vi "U3 DAC_Kevin_MFC_PID.vi"() -> ()   [LabVIEW 2016]
uses:
  OdorSensorArray/labview 2016 code/osa_global_save2.vi
  <vilib>/Utility/file.llb/Read From Spreadsheet File (DBL).vi
  <vilib>/measure/NI_MABase.lvlib
panel:
  out "Error  PID_Save":string
  out "error write":errorcluster
  in  "Save file":bool
  in  "data folder":path
  out "appended path":path
  out "PID_read":dbl(graph)
  out "AIN0":dbl format="%.6f"
  out "MFC I/O":cluster{"Value Read":dbl, "Value Read":dbl}(graph)
  out "AIN2":dbl format="%.6f"
  out "AIN1":dbl format="%.6f"
  in  "DAC0_type":enum16{"functional", "fixed", "read"}(ring)
  out "Array Size":i32
  out "Udate Array from File":sgl[](array[numeric])
  out "Waveform Chart":dbl(graph)
  in  "DAC0_fixed":dbl step=0.1 format="%.4f"
  out "Error DAC1,B":string
  out "error read":errorcluster
  in  "DAC1&DACB_fixed":dbl step=0.1 format="%.4f"
  in  "Update Interval (ms)":u32=20
  out "Error_DAC0":string
  in  "Function":u16(ring) items=["Sine Wave", "Triangle Wave", "Square Wave", "Sawtooth Wave"]
  in  "Min Voltage":dbl=0.5 min=0.0 max=5.0 step=0.1 format="%.2f"
  in  "Max Voltage":dbl=4.5 min=0.0 max=5.0 step=0.1 format="%.2f"
  in  "Frequency (Hz)":dbl=1.0 step=0.1 format="%.3f"
  in  "Stop":bool
  # "Updates DAC0 at the specified update interval in order to build time series waveforms.  The\nupdate interval is set to 20 ms by default, but can be set lower based on the execution times\ndiscussed in Section 3.1 of the U3 User's Guide.  Uses the first found U3.\n\nWith a software timed application such as this, you might be able to reduce timing jitter (caused\nby the operating system) by increasing the priority of this process (labview.exe) in Windows\nTask Manager."
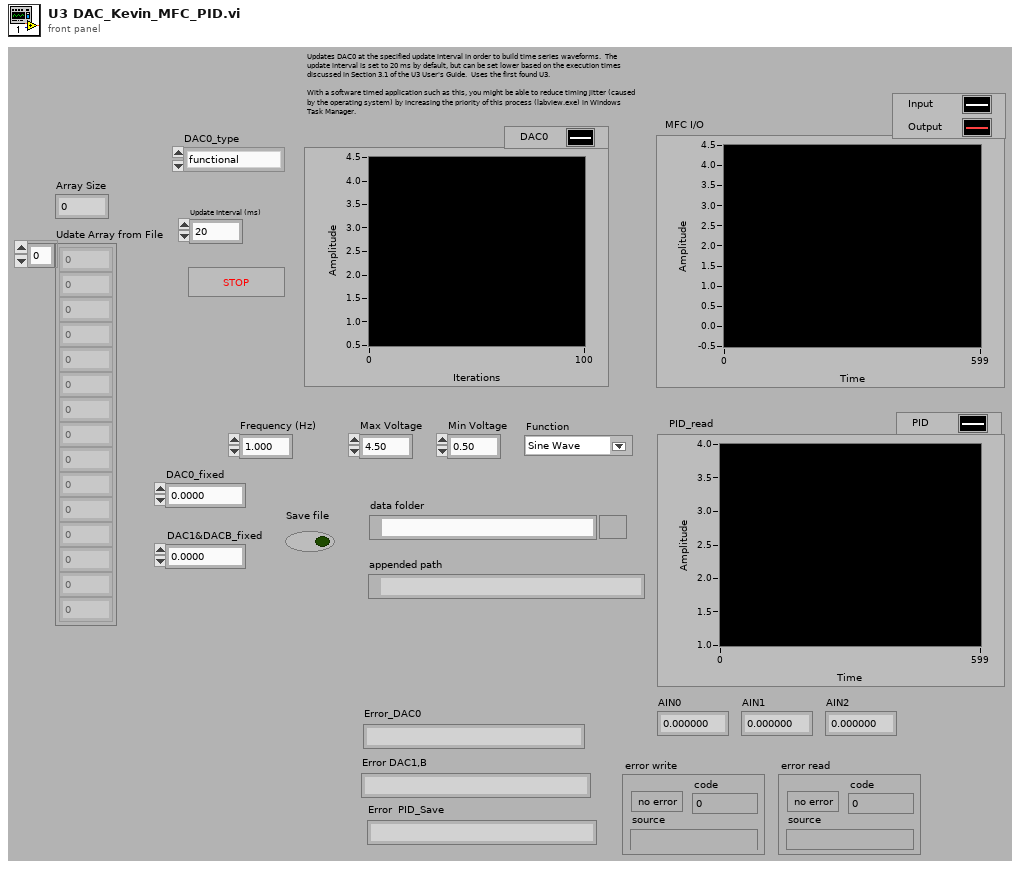
[diagram p1: front panel]
types:
  T1 = enum16{"open", "replace", "create", "open or create", "replace or create", "replace or create with confirmation"}
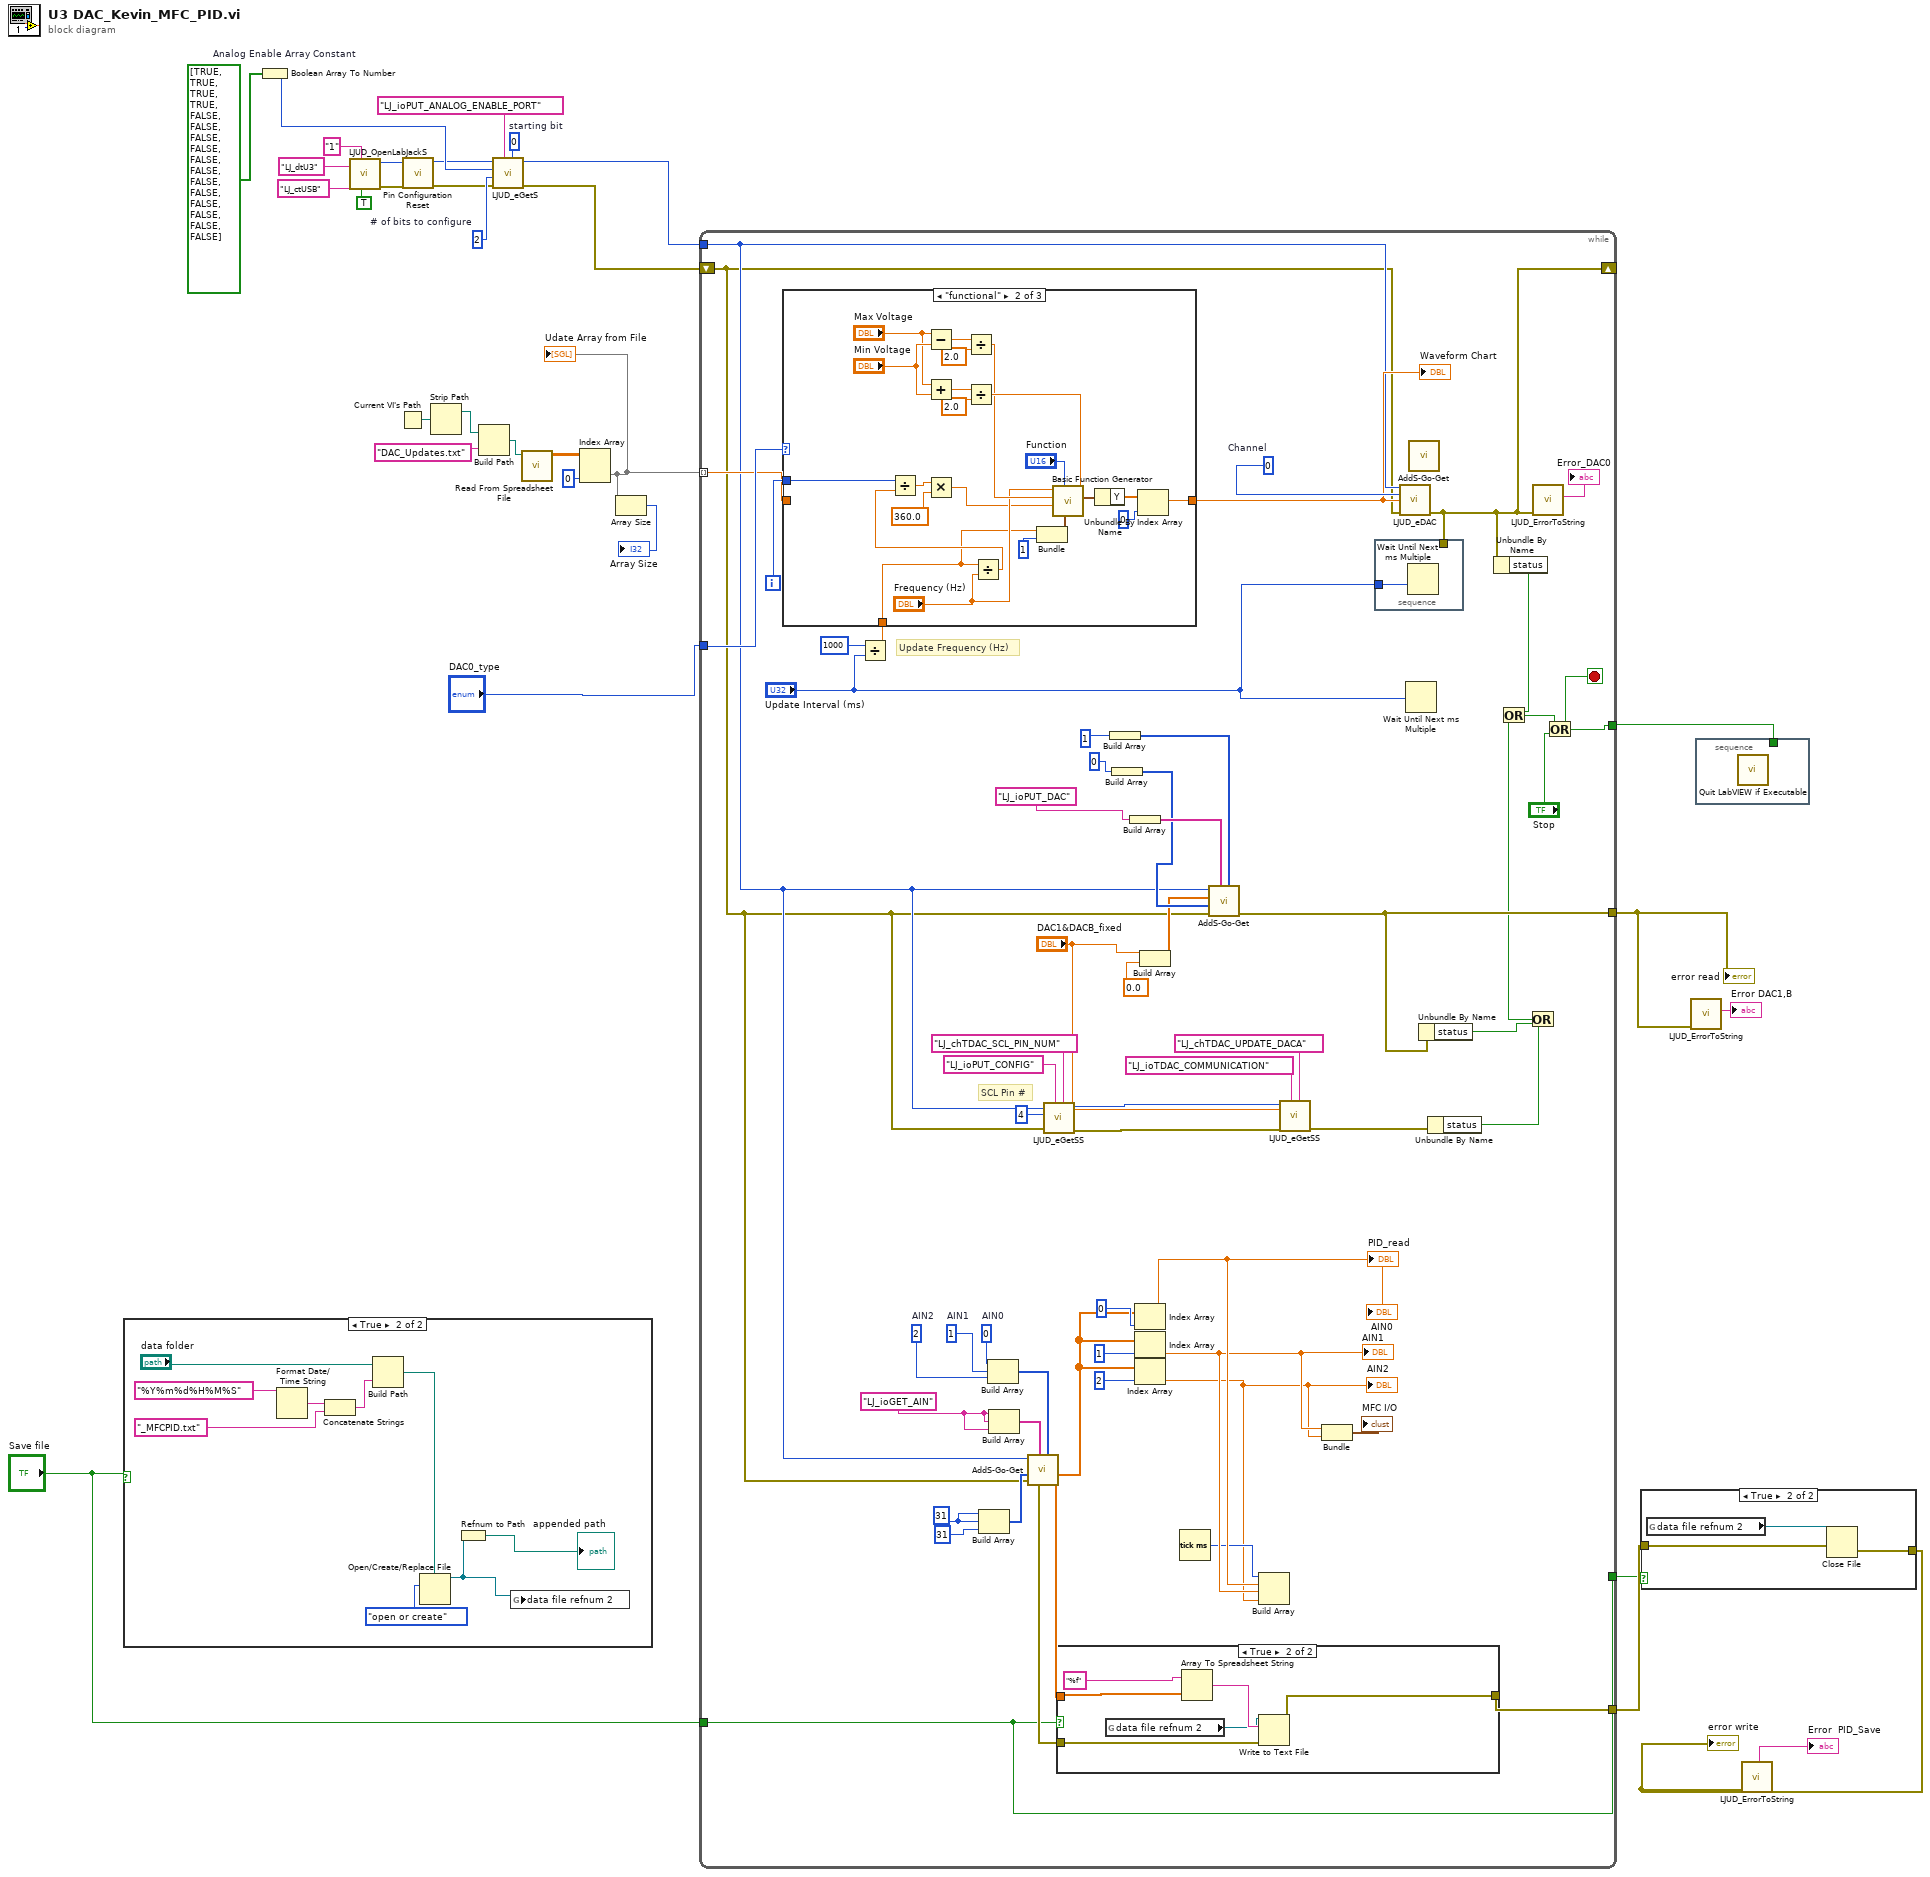
[diagram p0: block diagram]
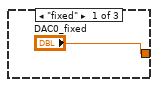
[diagram p5: hidden frame]
diagram:
  w11 = 2  # # of bits to configure
  w13 = 0  # starting bit
  w14 = bool[] [TRUE, TRUE, TRUE, TRUE, FALSE, FALSE, FALSE, FALSE, FALSE, FALSE, FALSE, FALSE, FALSE, FALSE, FALSE, FALSE]  # Analog Enable Array Constant
  n1 = case shown="True" "Save file" {
    frame False {
    }
    frame True {
      n2 = Format Date/Time String(time format string (%c)="%Y%m%d%H%M%S") -> (date/time string=w38:string)  [unwired: 2 in]
      n3 = Concatenate Strings(w38, "_MFCPID.txt") -> (w40:string)
      n4 = Build Path(base path="data folder", name or relative path=w40) -> (appended path=w34:path)
      n5 = Open/Create/Replace File(file path (use dialog)=w34, operation (0:open)=T1."open or create") -> (refnum out=w33:refnum<file>)  [unwired: 4 in, 2 out]
      n6 = Refnum to Path(1:w33) -> (0:→"appended path":path)
      n7 = global write "osa_global_save2.vi" "data file refnum 2"(w33) -> ()
    }
  }
  n8 = Boolean Array To Number(Boolean array=w14) -> (number=w10:u32)
  n9 = call "LJUD_OpenLabJackS.vi"("FirstFound"=TRUE, "Address"="1" ("DeviceType"), "ConnectionType"="LJ_ctUSB", "DeviceType"="LJ_dtU3") -> ("error out"=w15:errorcluster, "Handle"=w16:i32)  [unwired: 5 in, 1 out]
  n10 = Current VI's Path() -> (path=w24:path)
  n11 = call "Pin Configuration Reset.vi"("error in"=w15, "Handle In"=w16) -> ("error out"=w8:errorcluster, "Handle Out"=w9:i32)  [unwired: 8 in]
  n12 = Strip Path(path=w24) -> (stripped path=w23:path)  [unwired: 1 out]
  n13 = Build Path(base path=w23, name or relative path="DAC_Updates.txt" ("file path (dialog if empty)")) -> (appended path=w25:path)
  n14 = call "LJUD_eGetS.vi"("Channel"=w13, "IOType"="LJ_ioPUT_ANALOG_ENABLE_PORT", "error in"=w8, "x1"=w11, "Value Write"=w10, "Handle In"=w9) -> ("error out"=w6:errorcluster, "Handle Out"=w7:i32)  [unwired: 3 in, 1 out]
  n15 = call-poly <vilib>:"Read From Spreadsheet File.vi"("file path (dialog if empty)"=w25) -> ("all rows"=w29:dbl[][])  [unwired: 6 in, 4 out]
  n16 = Index Array(array=w29, index (col)=0 ("disabled index (col)")) -> (element=w22:dbl[])  [unwired: 1 in]
  "Udate Array from File" <- w22
  n17 = Array Size(array=w22) -> (size(s)=→"Array Size":i32)
  n18 = while {
    tunnel: w7 -> [w48]
    shift-left: w6 -> [w47]
    shift-right: [w95] -> _
    tunnel: [w81] -> w32
    tunnel: [w84] -> w30
    tunnel: "DAC0_type" -> [w79]
    tunnel: w22 -> [w78] mode=indexing
    tunnel: [w44] -> w5
    tunnel: "Save file" -> [w42]
    tunnel: [w42] -> w3
    i -> [w99]
    stop <- w81 stop-if-true
    w55 = 2  # AIN2
    w50 = 31 ("AIN0")
    w60 = 1  # AIN1
    w59 = 0  # AIN0
    w51 = "LJ_ioGET_AIN" ("IOType")
    w96 = 0  # Channel
    # "SCL Pin #"
    # "Update Frequency (Hz)"
    n19 = Divide(x=u32 1000, y="Update Interval (ms)") -> (x/y=w93:dbl)
    n20 = case shown="\"functional\"" w79 {
      tunnel: w99 -> [_ w129 _]
      tunnel: ["DAC0_fixed" w109 w130] -> w80
      tunnel: w93 -> [_ w108 _]
      tunnel: w78 -> [_ _ w130]
      frame "fixed" {
      }
      frame "functional" {
        n21 = Subtract(x="Max Voltage", y="Min Voltage") -> (x-y=w126:dbl)
        n22 = Add(x="Max Voltage", y="Min Voltage") -> (x+y=w123:dbl)
        n23 = Divide(x=w126, y=2.0) -> (x/y=w118:dbl)
        n24 = Divide(x=w123, y=2.0) -> (x/y=w119:dbl)
        n25 = Divide(x=w108, y="Frequency (Hz)") -> (x/y=w128:dbl)
        n26 = Divide(x=w129, y=w128) -> (x/y=w127:dbl)
        n27 = Multiply(x=w127, y=360.0) -> (x*y=w115:dbl)
        n28 = Bundle(w108, 1) -> (w113:cluster{dbl, i32})  [unwired: 1 in]
        n29 = call <vilib>:"Basic Function Generator.vi"("offset"=w119, "sampling info"=w113, "signal type"="Function", "phase"=w115, "amplitude"=w118, "frequency"="Frequency (Hz)") -> ("signal out"=w112:waveform(dbl))  [unwired: 3 in, 2 out]
        n30 = Unbundle By Name(w112) -> ("Y"=w111:dbl[])
        n31 = Index Array(array=w111, index=0 ("Index")) -> (element=w109:dbl)
      }
      frame "read" {
      }
    }
    "Waveform Chart" <- w80
    n32 = Build Array(w50, w50, 31 ("AIN1")) -> (w56:i32[])
    n33 = Build Array(w59, w60, w55) -> (w63:i32[])
    n34 = Build Array(w51, w51, w51) -> (w64:string[])
    n35 = call "AddS-Go-Get.vi"("Channels"=w63, "IOTypes"=w64, "error in"=w47, "x1"=w56, "Handle In"=w48) -> ("error out"=w45:errorcluster, "Values Read"=w43:dbl[])  [unwired: 4 in, 1 out]
    n36 = call "LJUD_eGetSS.vi"("Channel"="LJ_chTDAC_SCL_PIN_NUM", "IOType"="LJ_ioPUT_CONFIG", "error in"=w47, "Value Write"=4, "Handle In"=w48) -> ("error out"=w66:errorcluster, "Handle Out"=w67:i32)  [unwired: 4 in, 1 out]
    n37 = case shown="True" w42 {
      tunnel: w45 -> [w100 w105]
      tunnel: [w100 w104] -> w44
      tunnel: w43 -> [_ w101]
      frame False {
      }
      frame True {
        n38 = global read "osa_global_save2.vi" "data file refnum 2"() -> (w102:refnum<file>)
        n39 = Array To Spreadsheet String(array=w101, 3:"%f") -> (spreadsheet string=w103:string)  [unwired: 1 in]
        n40 = Write to Text File(file (use dialog)=w102, text=w103, error in=w105) -> (error out=w104:errorcluster)  [unwired: 1 in, 2 out]
      }
    }
    n41 = Build Array(1) -> (w91:i32[])
    n42 = Build Array(0) -> (w86:i32[])
    n43 = Build Array("LJ_ioPUT_DAC" ("IOType")) -> (w92:string[])
    n44 = Index Array(array=w43, index=0 ("Index")) -> (element=w53:dbl)
    "AIN0" <- w53
    "PID_read" <- w53
    n45 = Index Array(array=w43, index=1 ("Index")) -> (element=w52:dbl)
    "AIN1" <- w52
    n46 = Index Array(array=w43, index=2 ("Index")) -> (element=w46:dbl)
    "AIN2" <- w46
    n47 = Build Array("DAC1&DACB_fixed", 0.0 ("Input Element")) -> (w74:dbl[])
    n48 = Tick Count (ms)() -> (millisecond timer value=w49:u32)
    n49 = call "AddS-Go-Get.vi"("Channels"=w91, "IOTypes"=w92, "error in"=w47, "x1"=w86, "Values Write"=w74, "Handle In"=w48) -> ("error out"=w84:errorcluster)  [unwired: 3 in, 2 out]
    n50 = Build Array(w49, w53, w52, w46) -> ()  [unwired: 1 out]
    n51 = call "LJUD_eGetSS.vi"("Channel"="LJ_chTDAC_UPDATE_DACA", "IOType"="LJ_ioTDAC_COMMUNICATION", "error in"=w66, "Value Write"="DAC1&DACB_fixed", "Handle In"=w67) -> ("error out"=w68:errorcluster)  [unwired: 4 in, 2 out]
    n52 = Bundle("Value Read"=w52, "Value Read"=w46) -> (→"MFC I/O":cluster{"Value Read":dbl, "Value Read":dbl})  [unwired: 1 in]
    n53 = call "LJUD_eDAC.vi"("Handle In"=w48, "Channel"=w96, "Voltage"=w80, "error in"=w47) -> ("error out"=w95:errorcluster)  [unwired: 10 in, 1 out]
    n54 = stacked-sequence {
      tunnel: "Update Interval (ms)" -> [w131]
      tunnel: w95 -> [_]
      frame #0 {
        n55 = Wait Until Next ms Multiple(millisecond multiple=w131) -> ()  [unwired: 1 out]
      }
    }
    n56 = Wait Until Next ms Multiple(millisecond multiple="Update Interval (ms)") -> ()  [unwired: 1 out]
    n57 = call "AddS-Go-Get.vi"() -> ()  [unwired: 9 in, 3 out]
    n58 = Unbundle By Name(w84) -> ("status"=w71:bool)
    n59 = Unbundle By Name(w68) -> ("status"=w72:bool)
    n60 = Unbundle By Name(w95) -> ("status"=w83:bool)
    n61 = Or(x=w72, y=w71) -> (x .or. y?=w73:bool)
    n62 = Or(x=w83, y=w73) -> (x .or. y?=w82:bool)
    n63 = call "LJUD_ErrorToString.vi"("error in"=w95) -> ("String"=→"Error_DAC0":string)  [unwired: 10 in]
    n64 = Or(x=w82, y="Stop") -> (x .or. y?=w81:bool)
  }
  "error read" <- w30
  n65 = case shown="True" w3 {
    tunnel: w5 -> [w132 w135]
    tunnel: [w132 w134] -> w1
    frame False {
    }
    frame True {
      n66 = global read "osa_global_save2.vi" "data file refnum 2"() -> (w133:refnum<file>)
      n67 = Close File(refnum=w133, error in=w135) -> (error out=w134:errorcluster)  [unwired: 1 out]
    }
  }
  "error write" <- w1
  n68 = call "LJUD_ErrorToString.vi"("error in"=w30) -> ("String"=→"Error DAC1,B":string)  [unwired: 10 in]
  n69 = stacked-sequence {
    tunnel: w32 -> [_]
    frame #0 {
      n70 = call "Quit LabVIEW if Executable.vi"() -> ()  [unwired: 1 in]
    }
  }
  n71 = call "LJUD_ErrorToString.vi"("error in"=w1) -> ("String"=→"Error  PID_Save":string)  [unwired: 10 in]
